vi "Is Item Preloaded.vi"(7 "clear entries":bool, 8 "error in (no error)":errorcluster, 11 "Tag in":string) -> (0 "error out":errorcluster, 2 "replaced":bool, 3 "Tag out":string)   [LabVIEW 2020, in "DSF Core.lvlib"]
uses:
  DSF Core.lvlib
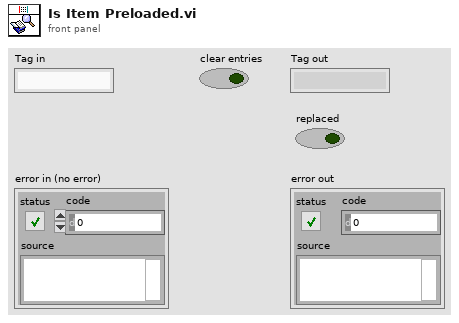
[diagram p1: front panel]
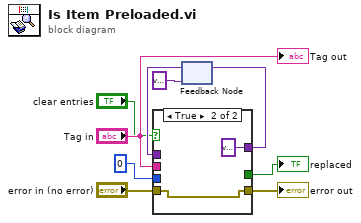
[diagram p0: block diagram]
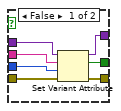
[diagram p2: hidden frame]
diagram:
  n1 = feedback #1(variant) -> (w3:variant)
  n2 = case shown="True" "clear entries" {
    tunnel: [w16 _] -> w9
    tunnel: 0 -> [w15 _]
    tunnel: "Tag in" -> [w14 _]
    tunnel: [w13 w17] -> w6
    tunnel: "error in (no error)" -> [w12 w17]
    tunnel: [w11 variant] -> w4
    tunnel: w3 -> [w10 _]
    frame False {
      n3 = Set Variant Attribute(Variant=w10, name=w14, value=w15, error in=w12) -> (Variant out=w11:variant, replaced=w16:bool, error out=w13:errorcluster)
    }
    frame True {
    }
  }
  "replaced" <- w9
  "error out" <- w6
  n4 = feedback-in #1(w4) -> ()
  "Tag out" <- "Tag in"
